vi "create client connector.vi"(8 "error in":errorcluster, 11 "engine context in":refnum<class "engine context.lvclass">) -> (0 "error out":errorcluster, 2 "client connector out":refnum<class "client connector.lvclass">)   [LabVIEW 2016, in "engine context.lvclass"]
uses:
  engine context.lvclass
  connection creator/client connector/client connector.lvclass
  engine context.lvclass/engine context.ctl
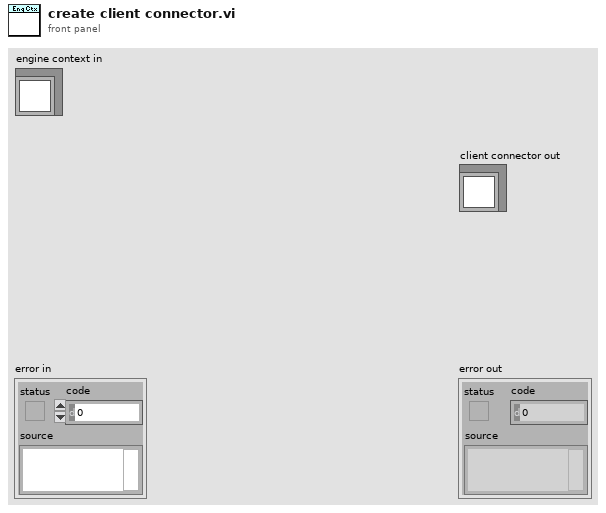
[diagram p1: front panel]
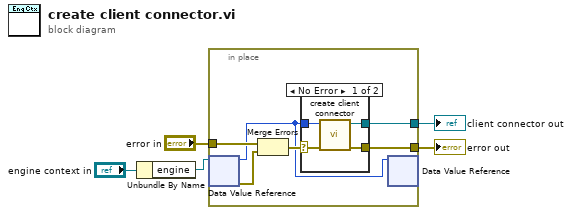
[diagram p0: block diagram]
diagram:
  n1 = Unbundle By Name("engine context in") -> ("engine"=w4:refnum<data-value>)
  n2 = in-place {
    in-place-border: "error in" -> [w11]
    in-place-border: [w8] -> w2
    in-place-border: [w7] -> w1
    n3 = in-place-dvr #1(w4) -> (w6:u64, w10:errorcluster)
    n4 = Merge Errors(w11, w10) -> (w9:errorcluster)
    n5 = case shown="No Error" w9 {
      selector: w9 -> [w14 w16]
      tunnel: w6 -> [w15 _]
      tunnel: [w12 w16] -> w8
      tunnel: [w13 _] -> w7
      frame No Error {
        n6 = call "create client connector.vi"("error in"=w14, "engine pointer"=w15) -> ("error out"=w12:errorcluster, "client connector out"=w13:refnum<class "client connector.lvclass">)  [unwired: 8 in]
      }
      frame Error {
      }
    }
    n7 = in-place-dvr #1(w6) -> ()  [unwired: 2 out]
  }
  "error out" <- w2
  "client connector out" <- w1
